vi "new_vi.vi"(11 "vi name":string) -> (3 "result":string)   [LabVIEW 2021]
panel:
  out "error out":errorcluster
  out "current time":timestamp
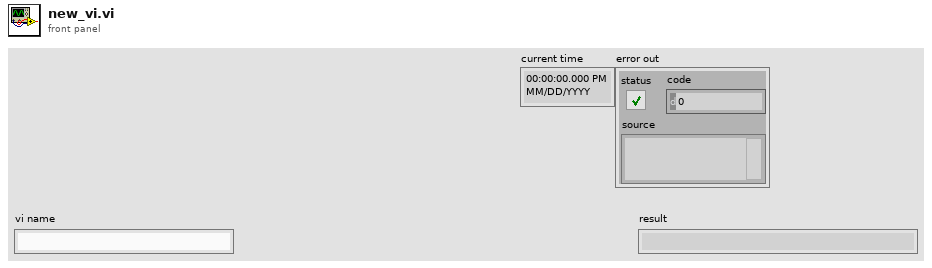
[diagram p1: front panel]
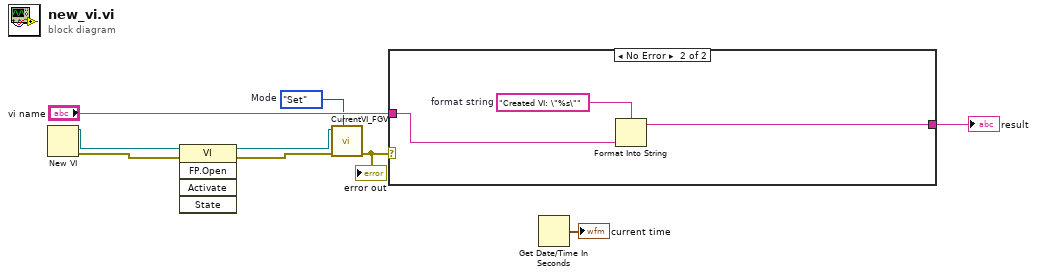
[diagram p0: block diagram]
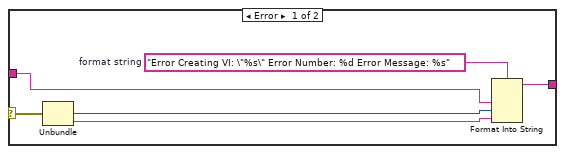
[diagram p2: hidden frame]
diagram:
  w1 = enum16{"Get", "Set"}."Set"  # Mode
  n1 = New VI() -> (0:w9:errorcluster, 3:w3:refnum<vi>)  [unwired: 7 in]
  n2 = invoke class="VI" method="FP.Open"(reference=w3, error in=w9) -> (reference out=w2:refnum<vi>, error out=w4:errorcluster)  [unwired: 3 in, 3 out]
  n3 = call "CurrentVI_FGV.vi"("Mode"=w1, "error in (no error)"=w4, "VI in"=w2) -> ("error out"=w8:errorcluster)  [unwired: 7 in, 1 out]
  "error out" <- w8
  n4 = case shown="No Error" w8 {
    selector: w8 -> [w13 _]
    tunnel: [w15 w17] -> w6
    tunnel: "vi name" -> [w10 w16]
    frame Error {
      w14 = "Error Creating VI: \"%s\" Error Number: %d Error Message: %s"  # format string
      n5 = Unbundle(w13) -> ("code"=w12:i32, "source"=w11:string)  [unwired: 1 out]
      n6 = Format Into String(format string=w14, w10, w12, w11) -> (resulting string=w15:string)  [unwired: 2 in, 1 out]
    }
    frame No Error {
      w18 = "Created VI: \"%s\""  # format string
      n7 = Format Into String(format string=w18, w16) -> (resulting string=w17:string)  [unwired: 2 in, 1 out]
    }
  }
  "result" <- w6
  n8 = Get Date/Time In Seconds() -> (seconds since 1Jan1904=→"current time":timestamp)
